vi "FPGA DDS SineGen IP.vi"(8 "Signal Amplitude (x 2^15)":u16=32768, 10 "Phase Shift":u32, 11 "Accumulator Increment":u32=100000) -> (1 "Accumulator Value":u32 format="%.3e", 2 "Cos output":i16, 3 "Sin output":i16)   [LabVIEW 2009]
doc: "This VI generates the next point on a DDS generated sine wave.\n\nThe accumulator increments to calculate the next phase value in the waveform. By varying the accumulator increment you control the frequency of the sine wave.\n\nThe accumulator phase value is used to select a value from the sine wave reference waveform stored in the Lookup Table VI. The waveformcan be p[hase shifted by specifying a non-zero phase shift value which is added to the accumulator phase. The output from the LUT is scaled using the AO Amplitude value."
uses:
  <vilib>/rvi/Arithmetic/AddSubMult/XNode/nirviSatArithmetic.xnode
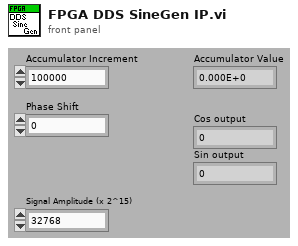
[diagram p1: front panel]
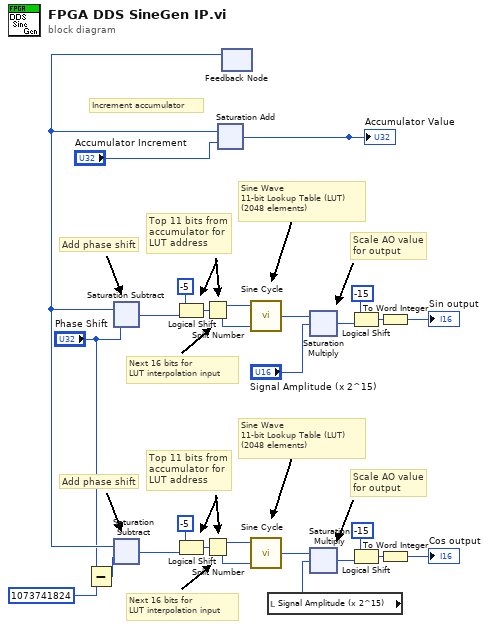
[diagram p0: block diagram]
diagram:
  # "Add phase shift"
  # "Scale AO value\nfor output"
  # "Next 16 bits for\nLUT interpolation input"
  # "Top 11 bits from \naccumulator for\nLUT address"
  # "Sine Wave \n11-bit Lookup Table (LUT)\n(2048 elements)"
  # "Add phase shift"
  # "Increment accumulator"
  # "Scale AO value\nfor output"
  # "Next 16 bits for\nLUT interpolation input"
  # "Top 11 bits from \naccumulator for\nLUT address"
  # "Sine Wave \n11-bit Lookup Table (LUT)\n(2048 elements)"
  n1 = Subtract(x="Phase Shift", y=u32 1073741824) -> (x-y=w3:u32)
  n2 = feedback #1() -> (w6:u32)  [unwired: 1 out]
  n3 = xnode "Saturation Subtract"("x"=w6, "y"="Phase Shift") -> ("x-y"=w17:u32)
  n4 = xnode "Saturation Subtract"("x"=w6, "y"=w3) -> ("x-y"=w7:u32)
  n5 = Logical Shift(y=-5, x=w17) -> (x << y=w21:u32)
  n6 = Logical Shift(y=-5, x=w7) -> (x << y=w10:u32)
  n7 = Split Number(x=w21) -> (hi(x)=w22:u16, lo(x)=w23:u16)
  n8 = Split Number(x=w10) -> (hi(x)=w11:u16, lo(x)=w12:u16)
  n9 = xnode ("Saturation Add")("x"=w6, "y"="Accumulator Increment") -> ("x+y"=w4:u32)
  "Accumulator Value" <- w4
  n10 = call "Sine Cycle"("address"=w22, "fractional index (x 2^16)"=w23) -> ("data out"=w24:i16)  [unwired: 7 out]
  n11 = call "Sine Cycle"("address"=w11, "fractional index (x 2^16)"=w12) -> ("data out"=w13:i16)  [unwired: 7 out]
  n12 = local read "Signal Amplitude (x 2^15)"() -> (w5:u16)
  n13 = xnode ("Saturation Multiply")("x"=w24, "y"="Signal Amplitude (x 2^15)") -> ("x*y"=w26:i32)
  n14 = xnode ("Saturation Multiply")("x"=w13, "y"=w5) -> ("x*y"=w14:i32)
  n15 = Logical Shift(y=-15, x=w26) -> (x << y=w28:i32)
  n16 = Logical Shift(y=-15, x=w14) -> (x << y=w16:i32)
  n17 = To Word Integer(number=w28) -> (16bit integer=→"Sin output":i16)
  n18 = To Word Integer(number=w16) -> (16bit integer=→"Cos output":i16)
